vi "asset.get_poly.vi"   [LabVIEW 2020, in "Nominal Client.lvclass"]
doc: "Returns one or more types.\nThis is a polymorphic function, that will accept a single RID or an array of RIDs."
uses:
  Nominal Client.lvclass
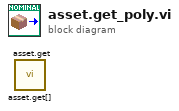
[diagram p0: block diagram]
diagram:
  n1 = call "asset.get[].vi"() -> ()  [unwired: 9 in, 3 out]
  n2 = call "asset.get.vi"() -> ()  [unwired: 9 in, 3 out]
